vi "one_scan.vi"(8 "error in (no error)":errorcluster, 11 "VISA Refnum in":refnum<visa-resource-name>) -> (0 "error out":errorcluster, 1 "PhiR Array":dbl[][](array[numeric]), 2 "XY Array":dbl[][](array[numeric]), 3 "VISA Refnum out":refnum<visa-resource-name>)   [LabVIEW 2014]
uses:
  <instrlib>/Hokuyo URG Series/Hokuyo URG Series.lvlib
types:
  T1 = cluster{"Magnitude":u16[], "Direction":fxp<+/-,16,8>[]}
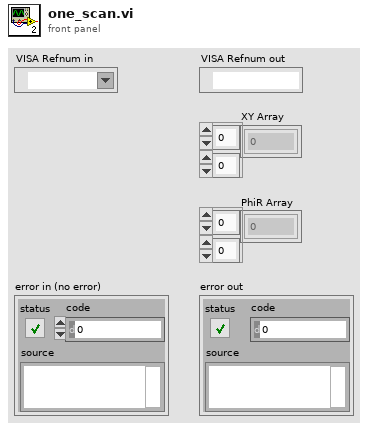
[diagram p1: front panel]
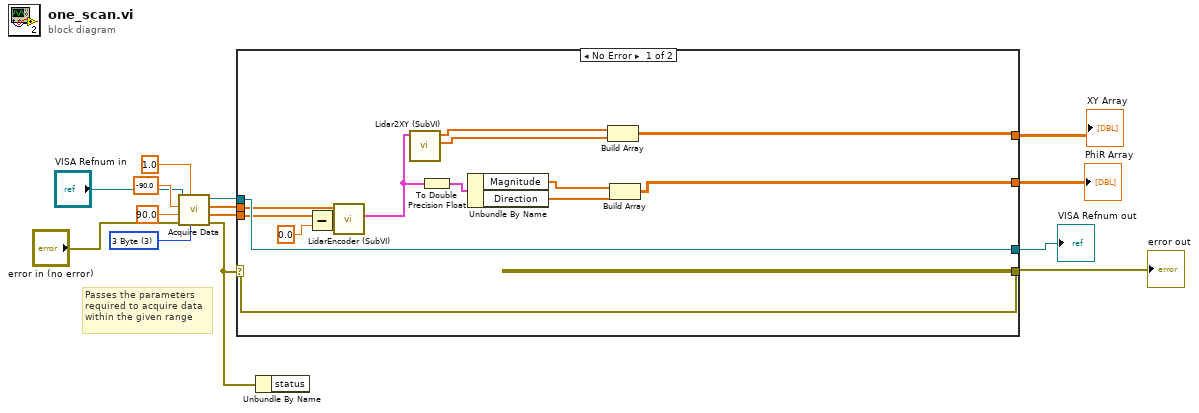
[diagram p0: block diagram]
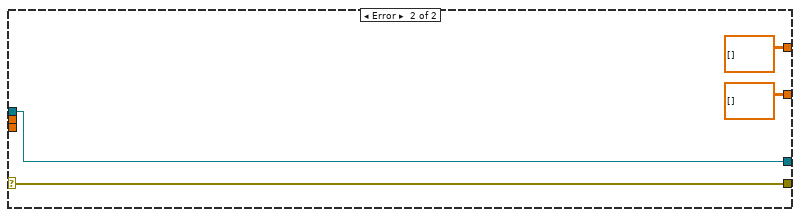
[diagram p2: hidden frame]
diagram:
  w12 = u16 3 items=["2 Byte"=2, "3 Byte"=3] ("Encoding Width")
  # "Passes the parameters\nrequired to acquire data\nwithin the given range"
  n1 = call <instrlib>:"Acquire Data.vi"("Data Encoding Width (3 Byte)"=w12, "Cluster Count (1)"=1.0 ("Cluster Count"), "error in (no error)"="error in (no error)", "End Point (120°)"=90.0 ("End Point"), "Start Point (-120°)"=-90.0 ("Start Point"), "VISA resource name"="VISA Refnum in") -> ("error out"=w8:errorcluster, "Direction"=w7:dbl[], "Magnitude"=w6:dbl[], "VISA resource name out"=w5:refnum<visa-resource-name>)  [unwired: 2 in]
  n2 = case shown="No Error" w8 {
    selector: w8 -> [w27 w32]
    tunnel: [w27 w32] -> w1
    tunnel: w5 -> [w28 w31]
    tunnel: [w28 w31] -> w2
    tunnel: w6 -> [w26 _]
    tunnel: w7 -> [w25 _]
    tunnel: [w16 dbl[][] []] -> w13
    tunnel: [w15 dbl[][] []] -> w14
    frame No Error {
      n3 = Subtract(x=w25, y=0.0) -> (x-y=w24:dbl[])
      n4 = call "LidarEncoder (SubVI).vi"("Direction"=w24, "Magnitude"=w26) -> ("Encoded"=w22:T1)  [unwired: 9 in]
      n5 = call "Lidar2XY (SubVI).vi"("Lidar"=w22) -> ("Y"=w17:dbl[], "X"=w18:dbl[])  [unwired: 9 in]
      n6 = To Double Precision Float(number=w22) -> (double precision float=w21:cluster{"Magnitude":dbl[], "Direction":dbl[]})
      n7 = Unbundle By Name(w21) -> ("Magnitude"=w20:dbl[], "Direction"=w19:dbl[])
      n8 = Build Array(w18, w17) -> (w15:dbl[][])
      n9 = Build Array(w20, w19) -> (w16:dbl[][])
    }
    frame Error {
    }
  }
  "XY Array" <- w14
  "PhiR Array" <- w13
  "VISA Refnum out" <- w2
  "error out" <- w1
  n10 = Unbundle By Name(w8) -> ()  [unwired: 1 out]
